vi "VI_Principale.vi"() -> ()   [LabVIEW 2023]
panel:
  out "Affichage":string="Mohamed"
  out "Login&Password":bool
  in  "Tab Control":enum32{"Page 1", "Page 2"}(tab)
  in  "First Name":string
  in  "Family Name":string
  in  "Password":string
  in  "Connect":bool
  in  "VALUE ---------->COLOR":bool
  in  "COLOR ---------->VALUE":bool
  in  "New code":bool
  in  "RESET":bool
  in  "stop Prg":bool
  in  "Tab Control SV-1":enum32{"Page 1", "Page 2"}(tab)
  in  "Tab Control Principal":enum32{"Page 1", "Page 2"}(tab)
  # "Convert Color Bands"
  # "Login"
  # "Value                                                 Color"
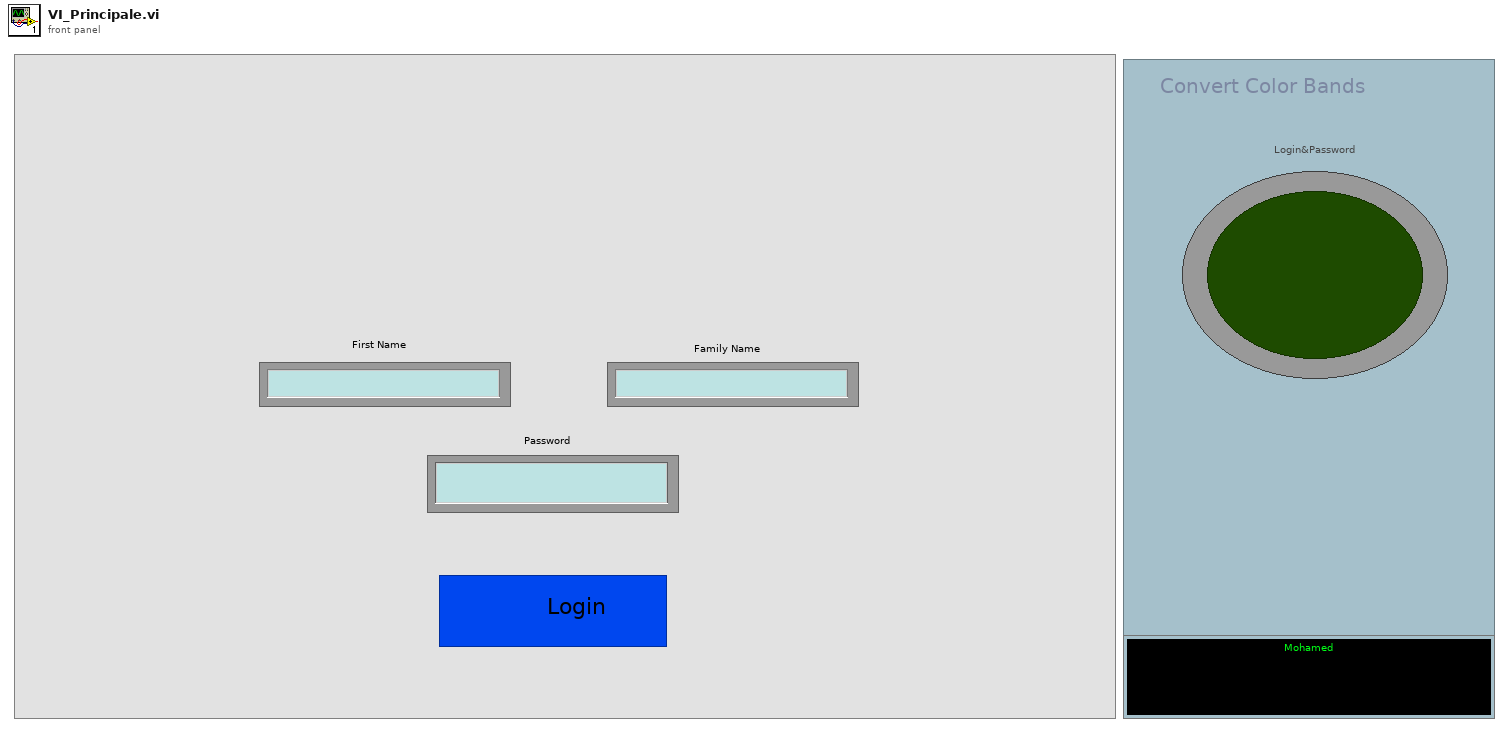
[diagram p1: front panel]
types:
  T1 = enum32{"Invalid", "Standard", "Closed", "Hidden", "Minimized", "Maximized"}
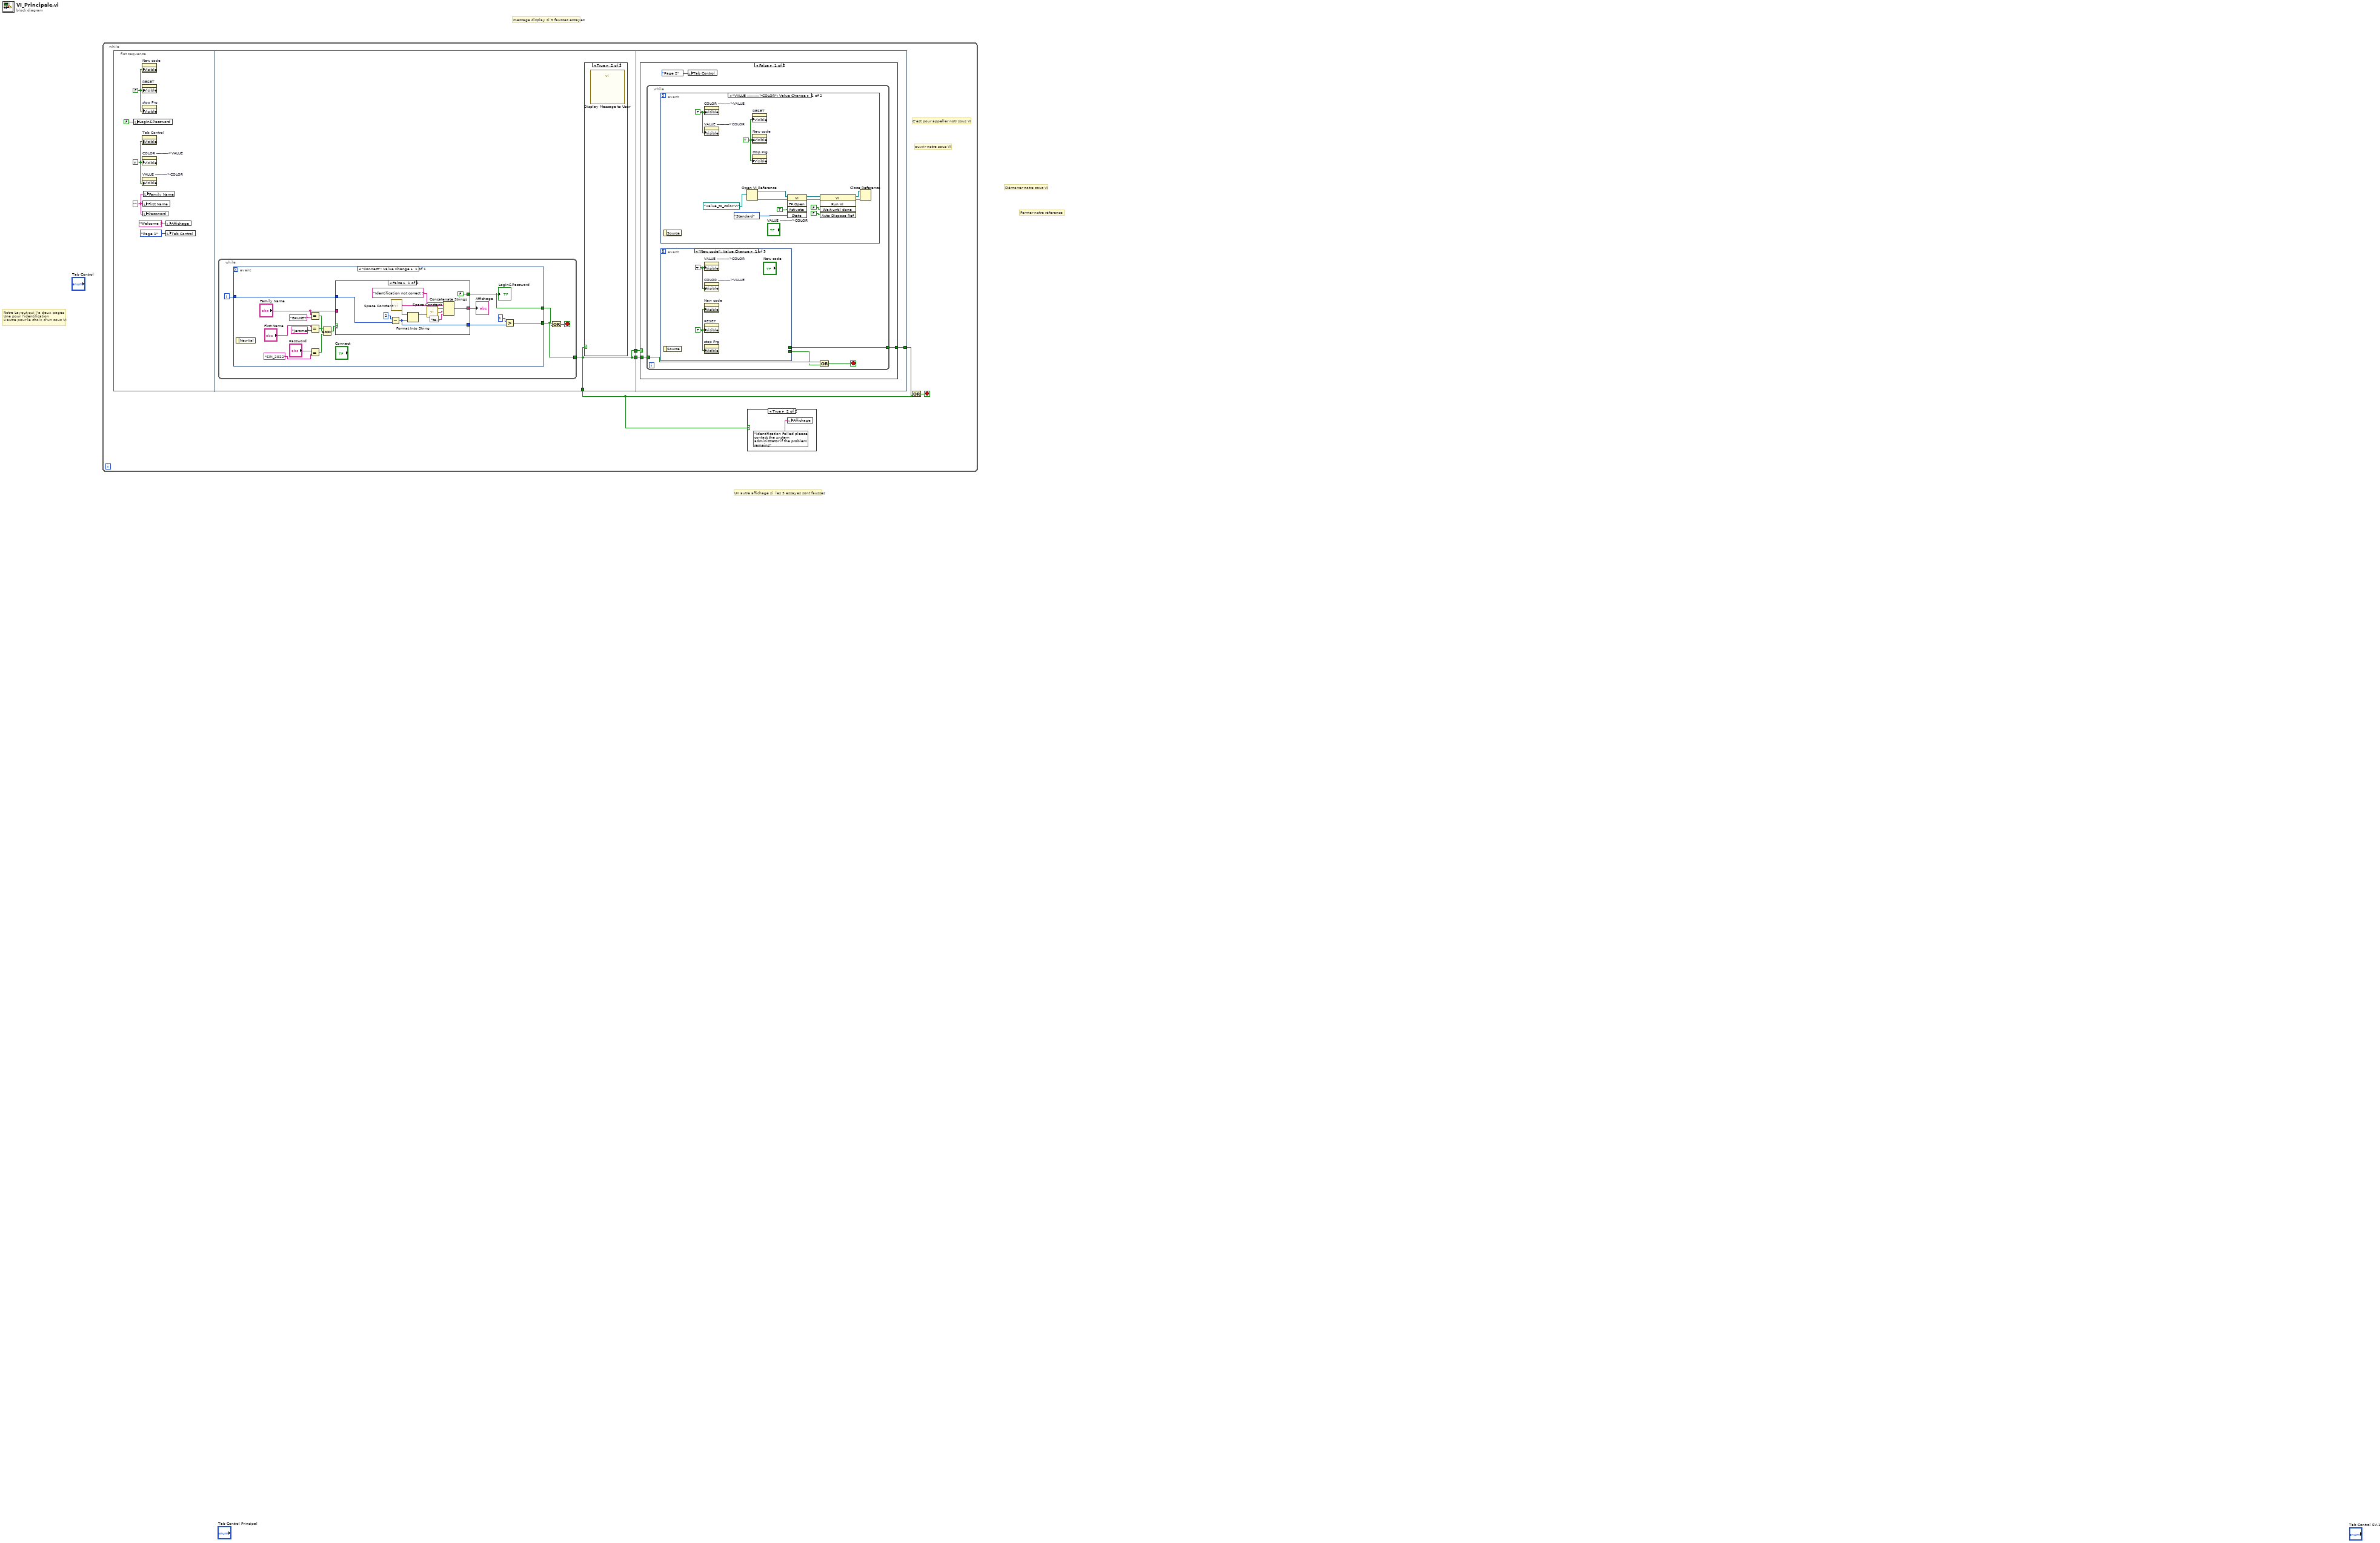
[diagram p0: block diagram]
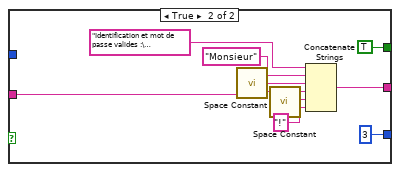
[diagram p4: hidden frame]
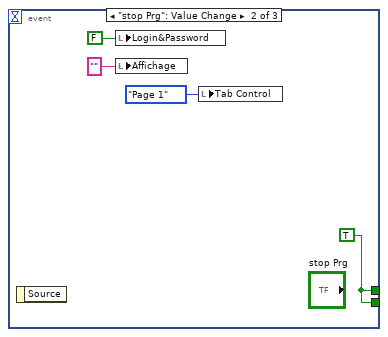
[diagram p5: hidden frame]
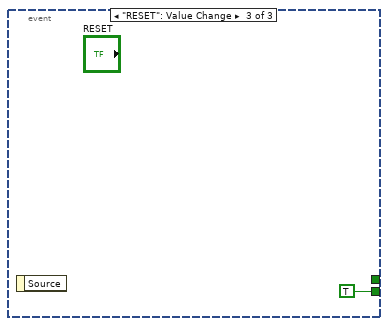
[diagram p6: hidden frame]
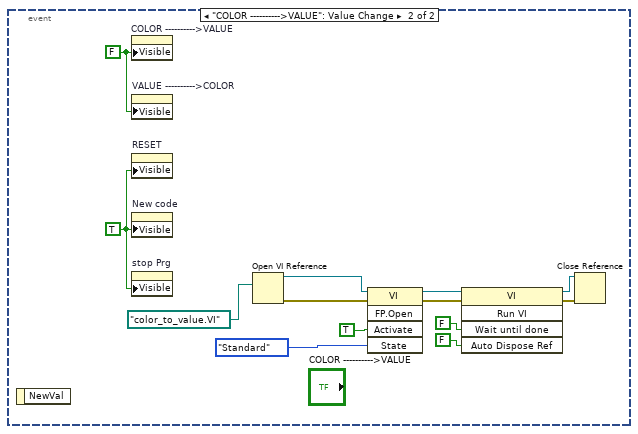
[diagram p7: hidden frame]
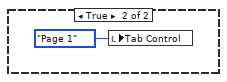
[diagram p8: hidden frame]
diagram:
  # "Un autre affichage si  les 3 essayes sont fausses"
  # "message display si 3 fausses essayes"
  # "Fermer notre réference"
  # "Démarrer notre sous VI"
  # "Notre Layout qui l'a deux pages\nUne pour l'identification\nL'autre pour le choix d'un sous VI"
  n1 = while {
    stop <- w3 stop-if-true
    # "ouvrir notre sous VI"
    # "C'est pour appeller notr sous VI"
    n2 = flat-sequence {
      tunnel: [w13] -> w5
      tunnel: [w13] -> w1
      tunnel: [w13] -> w4
      tunnel: w5 -> [w55]
      tunnel: w4 -> [w54]
      tunnel: [w53] -> w2
      frame #0 {
        w9 = FALSE ("Visible")
        w10 = TRUE ("Visible")
        w7 = "" ("Password")
        n3 = local write "Login&Password"(FALSE) -> ()
        n4 = property on="New code" class="Bool"("Visible"=w9) -> ()  [unwired: 2 in, 2 out]
        n5 = property on="RESET" class="Bool"("Visible"=w9) -> ()  [unwired: 2 in, 2 out]
        n6 = property on="stop Prg" class="Bool"("Visible"=w9) -> ()  [unwired: 2 in, 2 out]
        n7 = property on="Tab Control" class="TabCtl (strict)"("Visible"=w10) -> ()  [unwired: 2 in, 2 out]
        n8 = property on="COLOR ---------->VALUE" class="Bool"("Visible"=w10) -> ()  [unwired: 2 in, 2 out]
        n9 = property on="VALUE ---------->COLOR" class="Bool"("Visible"=w10) -> ()  [unwired: 2 in, 2 out]
        n10 = local write "First Name"(w7) -> ()
        n11 = local write "Password"(w7) -> ()
        n12 = local write "Family Name"(w7) -> ()
        n13 = local write "Affichage"("Welcome !" ("String")) -> ()
        n14 = local write "Tab Control"(enum32{"Page 1", "Page 2"}."Page 1" ("Tab Control")) -> ()
      }
      frame #1 {
        n15 = while {
          tunnel: [w16] -> w13
          i -> [w17]
          stop <- w15 stop-if-true
          n16 = event shown="[0] \"Connect\": Value Change" {
            selector: _ -> [_]
            dyn-events: _ -> [_]
            timeout: _ -> [_]
            tunnel: [w26] -> w14
            tunnel: w17 -> [w25]
            tunnel: [w23] -> w16
            event "Connect": Value Change {
              n17 = event-data() -> ()  [unwired: 1 in, 1 out]
              n18 = Equal?(x="Family Name", y="BRUNET") -> (x = y?=w32:bool)
              n19 = Equal?(x="First Name", y="Jerome") -> (x = y?=w31:bool)
              n20 = Equal?(x="Password", y="SPI_2022") -> (x = y?=w33:bool)
              n21 = Compound Arithmetic op=AND(w31, w32, w33) -> (w27:bool)
              n22 = case shown="False" w27 {
                tunnel: [FALSE TRUE] -> w26
                tunnel: [w36 w45] -> w20
                tunnel: [w39 3] -> w24
                tunnel: w25 -> [w41 _]
                tunnel: "Family Name" -> [_ w46]
                frame False {
                  n23 = Subtract(x=2, y=w41) -> (x-y=w39:i32)
                  n24 = call <vilib>:"Space Constant.vi"() -> ("String"=w38:string)
                  n25 = Format Into String(initial string=w38, w39) -> (resulting string=w37:string)  [unwired: 2 in, 1 out]
                  n26 = call <vilib>:"Space Constant.vi"() -> ("String"=w34:string)
                  n27 = Concatenate Strings("Identification not correct !", w38, w37, w34, "tentatives remaining") -> (w36:string)
                }
                frame True {
                  n28 = call <vilib>:"Space Constant.vi"() -> ("String"=w49:string)
                  n29 = call <vilib>:"Space Constant.vi"() -> ("String"=w48:string)
                  n30 = Concatenate Strings("Identification et mot de passe valides :\nBienvenu(e) ", "Monsieur", w49, w46, w48, "!") -> (w45:string)
                }
              }
              "Login&Password" <- w26
              "Affichage" <- w20
              n31 = Greater?(x=1, y=w24) -> (0:w23:bool)
            }
          }
          n32 = Compound Arithmetic op=OR(w16, w14) -> (w15:bool)
        }
        n33 = case shown="True" w13 {
          frame False {
          }
          frame True {
            n34 = call "Display Message to User"() -> ()  [unwired: 10 in, 2 out]
          }
        }
      }
      frame #2 {
        n35 = case shown="False" w55 {
          tunnel: w54 -> [w58 _]
          tunnel: [w57 _] -> w53
          frame False {
            n36 = while {
              tunnel: w58 -> [w62]
              tunnel: [w59] -> w57
              stop <- w61 stop-if-true
              n37 = event shown="[0] \"VALUE ---------->COLOR\": Value Change" {
                selector: _ -> [_ _]
                dyn-events: _ -> [_ _]
                timeout: _ -> [_ _]
                event "VALUE ---------->COLOR": Value Change {
                  w71 = FALSE ("Visible")
                  w70 = TRUE ("Visible")
                  n38 = event-data() -> ()  [unwired: 1 in, 1 out]
                  n39 = property on="COLOR ---------->VALUE" class="Bool"("Visible"=w71) -> ()  [unwired: 2 in, 2 out]
                  n40 = property on="VALUE ---------->COLOR" class="Bool"("Visible"=w71) -> ()  [unwired: 2 in, 2 out]
                  n41 = Open VI Reference(vi path=path "value_to_color.VI") -> (vi reference=w79:refnum<vi>, error out=w78:errorcluster)  [unwired: 5 in]
                  n42 = property on="RESET" class="Bool"("Visible"=w70) -> ()  [unwired: 2 in, 2 out]
                  n43 = property on="New code" class="Bool"("Visible"=w70) -> ()  [unwired: 2 in, 2 out]
                  n44 = property on="stop Prg" class="Bool"("Visible"=w70) -> ()  [unwired: 2 in, 2 out]
                  n45 = invoke class="VI" method="FP.Open"(reference=w79, error in=w78, "Activate"=TRUE ("Activate?"), "State"=T1."Standard") -> (reference out=w81:refnum<vi>, error out=w80:errorcluster)  [unwired: 1 in, 3 out]
                  n46 = invoke class="VI" method="Run VI"(reference=w81, error in=w80, "Wait until done"=FALSE ("Wait Until Done"), "Auto Dispose Ref"=FALSE ("Auto Dispose Reference")) -> (reference out=w77:refnum<vi>, error out=w76:errorcluster)  [unwired: 1 in, 3 out]
                  n47 = Close Reference(reference=w77, error in (no error)=w76) -> ()  [unwired: 1 out]
                }
                event "COLOR ---------->VALUE": Value Change {
                  w83 = TRUE ("Visible")
                  w89 = FALSE ("Visible")
                  n48 = event-data() -> ()  [unwired: 1 in, 1 out]
                  n49 = property on="COLOR ---------->VALUE" class="Bool"("Visible"=w89) -> ()  [unwired: 2 in, 2 out]
                  n50 = property on="VALUE ---------->COLOR" class="Bool"("Visible"=w89) -> ()  [unwired: 2 in, 2 out]
                  n51 = property on="RESET" class="Bool"("Visible"=w83) -> ()  [unwired: 2 in, 2 out]
                  n52 = property on="New code" class="Bool"("Visible"=w83) -> ()  [unwired: 2 in, 2 out]
                  n53 = property on="stop Prg" class="Bool"("Visible"=w83) -> ()  [unwired: 2 in, 2 out]
                  n54 = Open VI Reference(vi path=path "color_to_value.VI") -> (vi reference=w92:refnum<vi>, error out=w93:errorcluster)  [unwired: 5 in]
                  n55 = invoke class="VI" method="FP.Open"(reference=w92, error in=w93, "Activate"=TRUE ("Activate?"), "State"=T1."Standard") -> (reference out=w90:refnum<vi>, error out=w91:errorcluster)  [unwired: 1 in, 3 out]
                  n56 = invoke class="VI" method="Run VI"(reference=w90, error in=w91, "Wait until done"=FALSE ("Wait Until Done"), "Auto Dispose Ref"=FALSE ("Auto Dispose Reference")) -> (reference out=w94:refnum<vi>, error out=w95:errorcluster)  [unwired: 1 in, 3 out]
                  n57 = Close Reference(reference=w94, error in (no error)=w95) -> ()  [unwired: 1 out]
                }
              }
              n58 = event shown="[0] \"New code\": Value Change" {
                selector: _ -> [_ _ _]
                dyn-events: _ -> [_ _ _]
                timeout: _ -> [_ _ _]
                tunnel: [_ w68 TRUE] -> w60
                tunnel: [_ w68 _] -> w59
                event "New code": Value Change {
                  w63 = FALSE ("Visible")
                  w64 = TRUE ("Visible")
                  n59 = event-data() -> ()  [unwired: 1 in, 1 out]
                  n60 = property on="VALUE ---------->COLOR" class="Bool"("Visible"=w64) -> ()  [unwired: 2 in, 2 out]
                  n61 = property on="COLOR ---------->VALUE" class="Bool"("Visible"=w64) -> ()  [unwired: 2 in, 2 out]
                  n62 = property on="New code" class="Bool"("Visible"=w63) -> ()  [unwired: 2 in, 2 out]
                  n63 = property on="RESET" class="Bool"("Visible"=w63) -> ()  [unwired: 2 in, 2 out]
                  n64 = property on="stop Prg" class="Bool"("Visible"=w63) -> ()  [unwired: 2 in, 2 out]
                }
                event "stop Prg": Value Change {
                  w68 = TRUE
                  n65 = event-data() -> ()  [unwired: 1 in, 1 out]
                  n66 = local write "Login&Password"(FALSE ("lampa")) -> ()
                  n67 = local write "Affichage"("" ("Affichage")) -> ()
                  n68 = local write "Tab Control"(enum32{"Page 1", "Page 2"}."Page 1" ("Tab Control")) -> ()
                }
                event "RESET": Value Change {
                  n69 = event-data() -> ()  [unwired: 1 in, 1 out]
                }
              }
              n70 = Compound Arithmetic op=OR(w62, w60) -> (w61:bool)
            }
            n71 = local write "Tab Control"(enum32{"Page 1", "Page 2"}."Page 2" ("Tab Control")) -> ()
          }
          frame True {
            n72 = local write "Tab Control"(enum32{"Page 1", "Page 2", "Page 3"}."Page 1" ("Tab Control")) -> ()
          }
        }
      }
    }
    n73 = case shown="True" w1 {
      frame False {
      }
      frame True {
        n74 = local write "Affichage"("Identification Failed please contact the system administrator if the problem remains" ("Affichage")) -> ()
      }
    }
    n75 = Compound Arithmetic op=OR(w1, w2) -> (w3:bool)
  }
